vi "Execute.vi"(6 "Index [-1]":i32=-1, 7 "Composite Object":refnum<class "CConfig Object.lvclass">, 8 "error in (no error)":errorcluster, 9 "Results":string[][](array[string]), 11 "Config Query in":refnum<class "Composite Query.lvclass">) -> (0 "error out":errorcluster, 1 "Results":string[][](array[string]), 2 "Result":bool, 3 "Config Query out":refnum<class "Composite Query.lvclass">, 4 "Index":i32, 5 "Composite Object":refnum<class "CConfig Object.lvclass">)   [LabVIEW 2013, in "Composite Query.lvclass"]
doc: "Copyright 2018, Carya Automatisering, Wiebe Walstra."
uses:
  Composite Query.lvclass
  CConfig Object.lvclass
  Composite Query.lvclass/Composite Query.ctl
  CConfig Query.lvclass
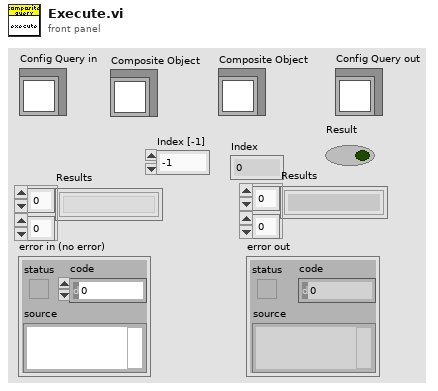
[diagram p1: front panel]
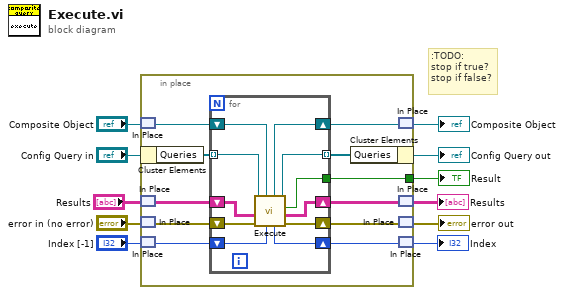
[diagram p0: block diagram]
diagram:
  # ":TODO:\nstop if true?\nstop if false?"
  n1 = in-place {
    in-place-border: [w22] -> w11
    n2 = in-place-match #1("Composite Object") -> (w17:refnum<class "CConfig Object.lvclass">)
    n3 = in-place-cluster #2("Config Query in") -> ("Queries"=w21:refnum<class "CConfig Query.lvclass">[])
    n4 = in-place-match #3("Results") -> (w19:string[][])
    n5 = in-place-match #4("error in (no error)") -> (w15:errorcluster)
    n6 = in-place-match #5("Index [-1]") -> (w13:i32)
    n7 = for {
      tunnel: [w28] -> w22
      tunnel: w21 -> [w27] mode=indexing
      tunnel: [w26] -> w20 mode=indexing
      shift-right: [w29] -> w16
      shift-left: w17 -> [w30]
      shift-right: [w32] -> w14
      shift-left: w15 -> [w33]
      shift-right: [w25] -> w12
      shift-left: w13 -> [w31]
      shift-right: [w24] -> w18
      shift-left: w19 -> [w23]
      n8 = call-dynamic "Execute.vi"("Index [-1]"=w31, "Composite Object"=w30, "error in (no error)"=w33, "Results"=w23, "Config Query in"=w27) -> ("error out"=w32:errorcluster, "Results"=w24:string[][], "Result"=w28:bool, "Config Query out"=w26:refnum<class "CConfig Query.lvclass">, "Index"=w25:i32, "Composite Object"=w29:refnum<class "CConfig Object.lvclass">)  [unwired: 1 in]
    }
    n9 = in-place-cluster #2("Queries"=w20) -> (→"Config Query out":refnum<class "Composite Query.lvclass">)
    n10 = in-place-match #1(w16) -> (→"Composite Object":refnum<class "CConfig Object.lvclass">)
    n11 = in-place-match #3(w18) -> (→"Results":string[][])
    n12 = in-place-match #4(w14) -> (→"error out":errorcluster)
    n13 = in-place-match #5(w12) -> (→"Index":i32)
  }
  "Result" <- w11
